vi "2039_2017vis GetCenterPosition.vi"(1 "Image Size":cluster{"X Resolution":i32, "Y Resolution":i32}, 2 "Objects":T1(array[cluster]) {"Aspect Ratio" format="%.2f"; "Orientation" format="%.2f"; "Area" format="%.2f"; "Object Center"."Y" format="%.2f"; "Object Center"."X" format="%.2f"}) -> (0 "Center X Offset":i32)   [LabVIEW 2016, in "2039lib.lvlib"]
uses:
  2039lib.lvlib
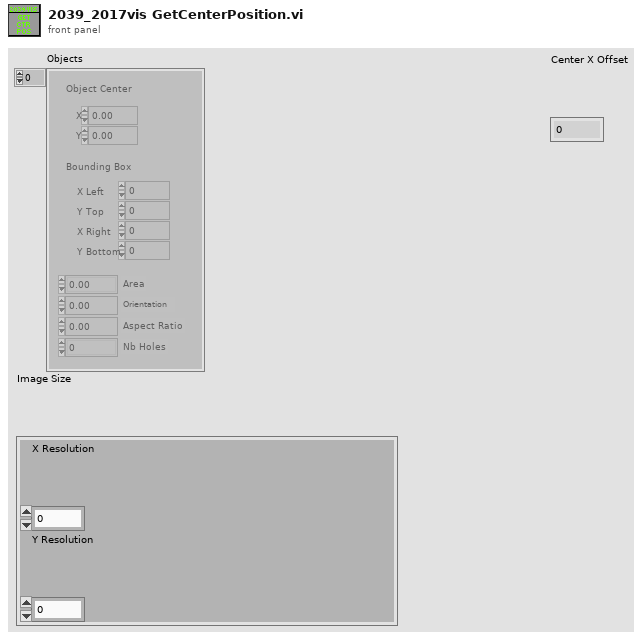
[diagram p1: front panel]
types:
  T1 = cluster{"Object Center":cluster{"X":sgl, "Y":sgl}, "Bounding Box":cluster{"X Left":i32, "Y Top":i32, "X Right":i32, "Y Bottom":i32}, "Area":sgl, "Orientation":sgl, "Aspect Ratio":sgl, "Nb Holes":i32}[]
  T2 = cluster{"Object Center":cluster{"X":sgl, "Y":sgl}, "Bounding Box":cluster{"X Left":i32, "Y Top":i32, "X Right":i32, "Y Bottom":i32}, "Area":sgl, "Orientation":sgl, "Aspect Ratio":sgl, "Nb Holes":i32}
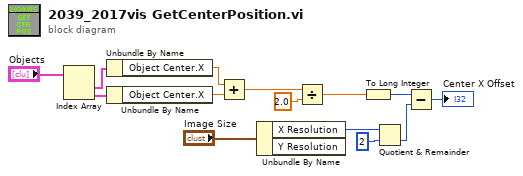
[diagram p0: block diagram]
diagram:
  n1 = Index Array(array="Objects") -> (element #1=w13:T2, element #2=w12:T2)  [unwired: 2 in]
  n2 = Unbundle By Name(w13) -> ("Object Center.X"=w11:sgl)
  n3 = Unbundle By Name(w12) -> ("Object Center.X"=w10:sgl)
  n4 = Add(x=w11, y=w10) -> (x+y=w9:sgl)
  n5 = Unbundle By Name("Image Size") -> ("X Resolution"=w6:i32)  [unwired: 1 out]
  n6 = Divide(x=w9, y=2.0) -> (x/y=w3:dbl)
  n7 = To Long Integer(number=w3) -> (32bit integer=w2:i32)
  n8 = Quotient & Remainder(x=w6, y=2) -> (floor(x/y)=w4:i32)  [unwired: 1 out]
  n9 = Subtract(x=w2, y=w4) -> (x-y=→"Center X Offset":i32)
